vi "Stop Event Handler.vi"(8 "error in (no error)":errorcluster, 11 "ActorAutoRegistration in":refnum<class "ActorAutoRegistration.lvclass">) -> (0 "error out":errorcluster)   [LabVIEW 2015, in "ActorAutoRegistration.lvlib" / "ActorAutoRegistration.lvclass"]
uses:
  ActorAutoRegistration.lvclass
  ActorAutoRegistration.lvclass/ActorAutoRegistration.ctl
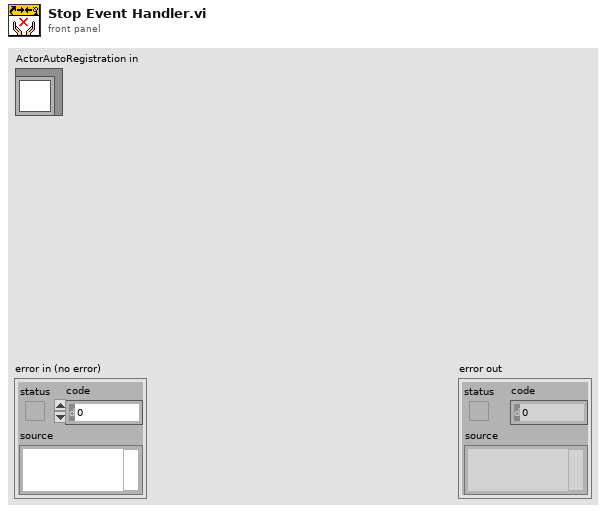
[diagram p1: front panel]
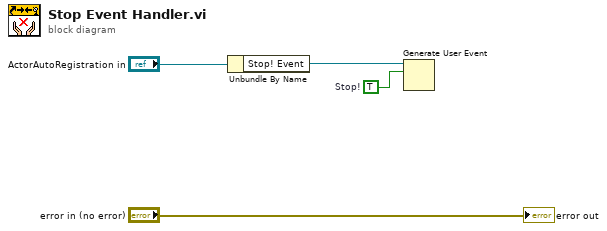
[diagram p0: block diagram]
diagram:
  w1 = TRUE  # Stop!
  n1 = Unbundle By Name("ActorAutoRegistration in") -> ("Stop! Event"=w2:refnum<user-event>)
  n2 = Generate User Event(user event=w2, event data cluster=w1) -> ()  [unwired: 2 in, 2 out]
  "error out" <- "error in (no error)"
